vi "AuthenticationTest.vi"(8 "error in (no error)":errorcluster) -> (0 "error out":errorcluster, 3 "Match?":bool)   [LabVIEW 2016, in "User Interface.lvlib"]
uses:
  User Interface.lvlib
  Authentication State.ctl
  Database/Database.lvlib
  Database/Class/DB/Credential.ctl
  Action log.ctl
panel:
  out "Time 2":string="Authentication"
  out "Msg Out":string
  in  "Password":string
  in  "Username":string(combo)
  in  "User Level":string(combo)
  in  "Cancel":bool
  in  "Delete":bool
  in  "Add":bool
  in  "Edit":bool
  in  "Authentication Tab":enum32{"User", "Edit User"}(tab)
  in  "User Name":string(combo)
  in  "Password":string
  in  "Log":bool
  out "Time":string="Sat  8/3/2019  8:10:44 PM"
  in  "Update":bool
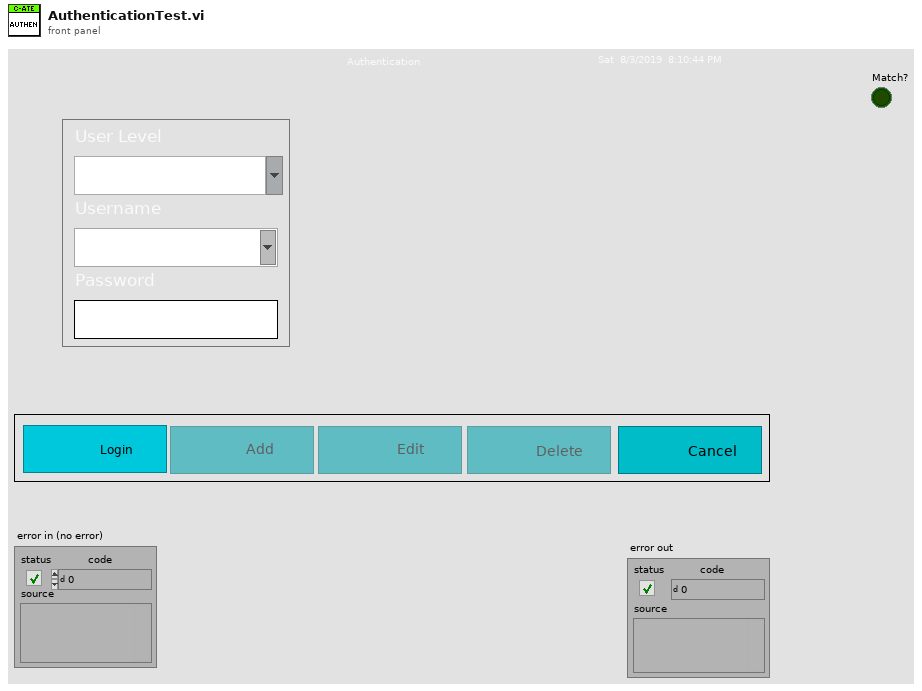
[diagram p1: front panel]
types:
  T1 = typedef "User Interface.lvlib/Authentication State.ctl" = enum16{"Initialize", "Main", "Add User", "Delete User", "Close"}
  T2 = typedef "User Interface.lvlib/Action log.ctl" = enum16{"Init", "Read", "Write", "Close"}
  T3 = typedef "Database.lvlib/Credential.ctl" = cluster{"User Level":string, "User Name":string, "Password":string}
  T4 = enum8{"Enabled", "Disabled", "Disabled and Grayed Out"}
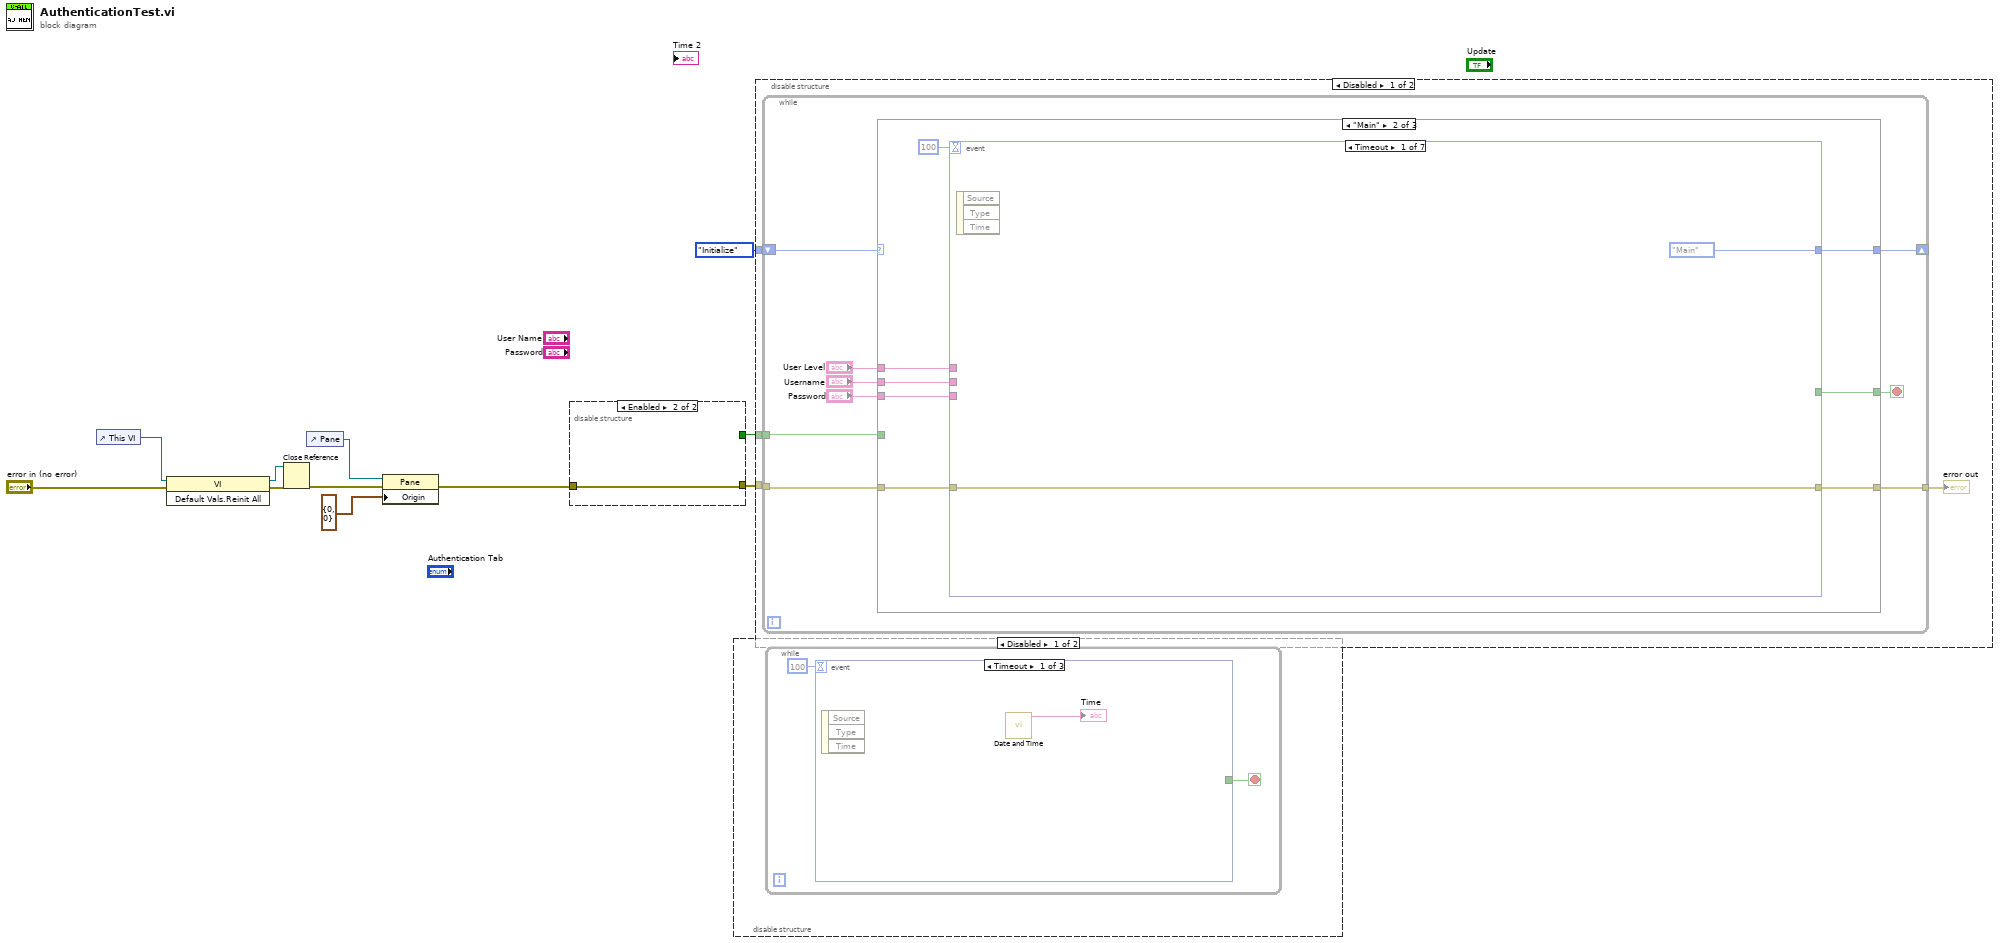
[diagram p0: block diagram]
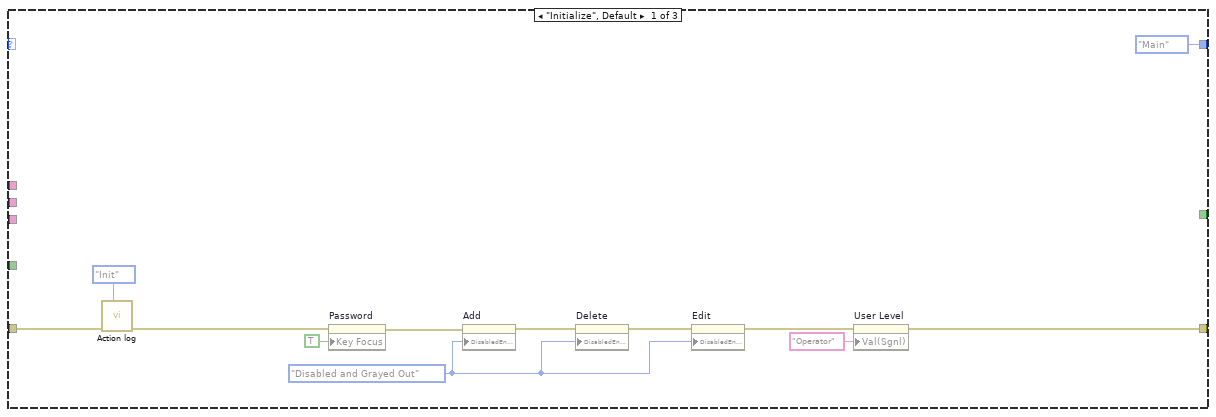
[diagram p2: hidden frame]
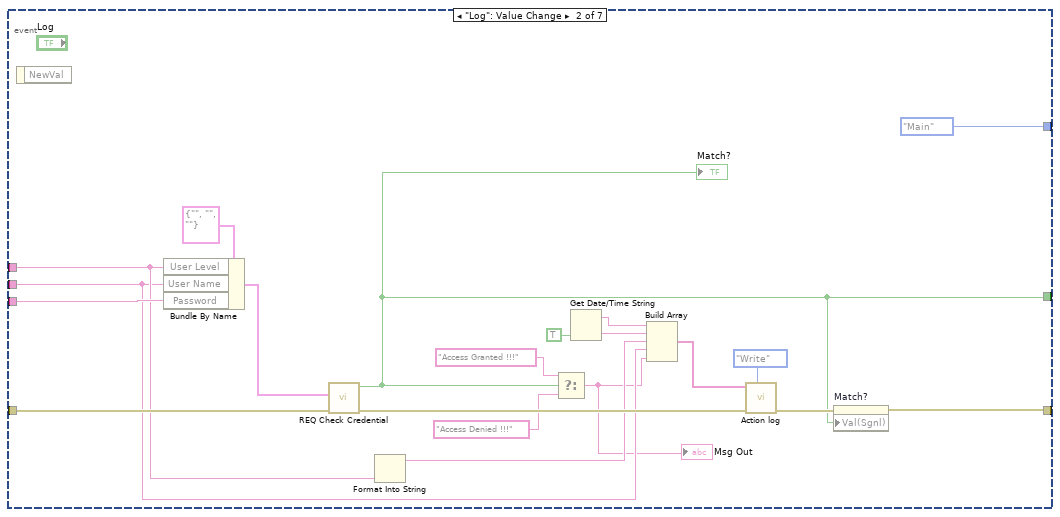
[diagram p3: hidden frame]
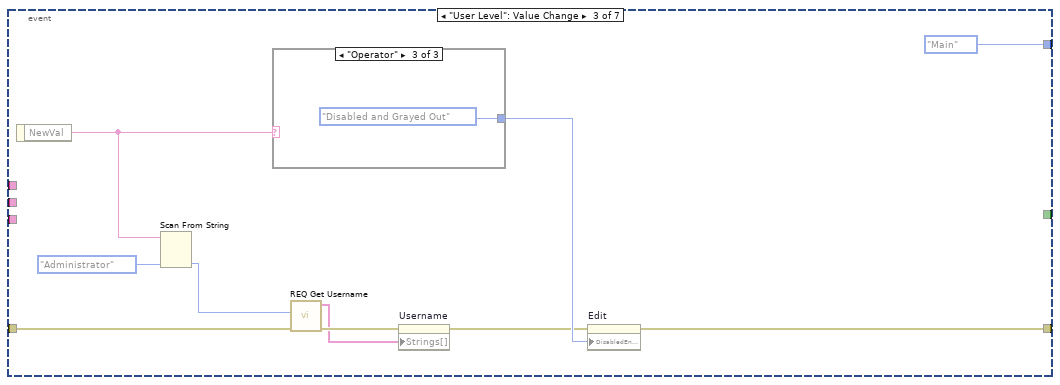
[diagram p4: hidden frame]
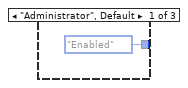
[diagram p5: hidden frame]
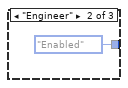
[diagram p6: hidden frame]
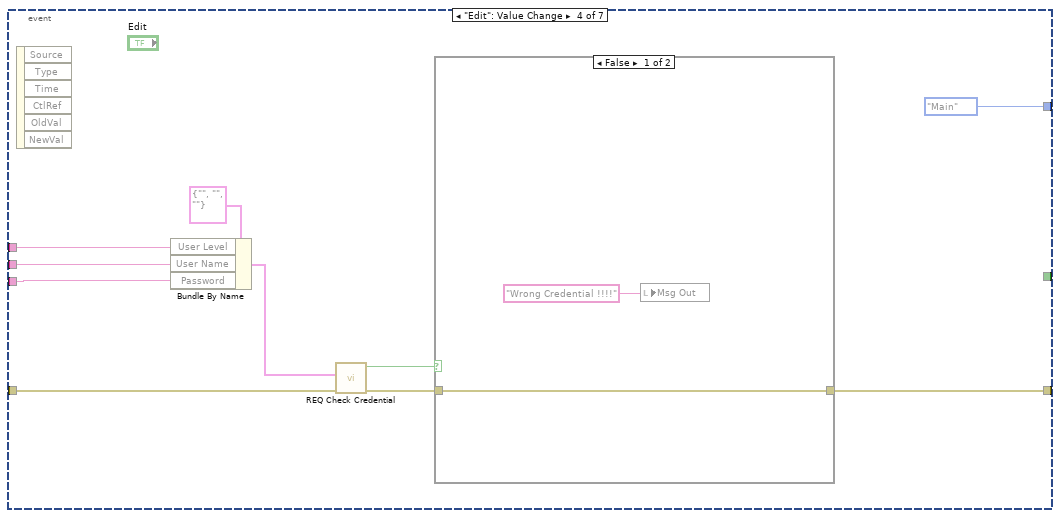
[diagram p7: hidden frame]
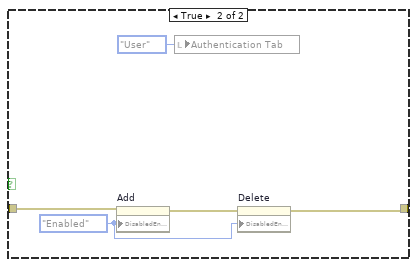
[diagram p8: hidden frame]
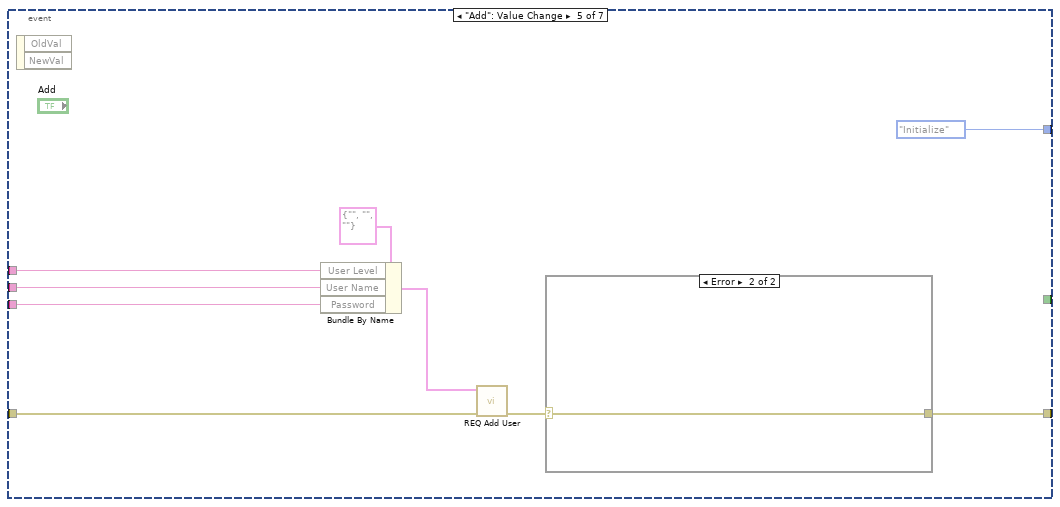
[diagram p9: hidden frame]
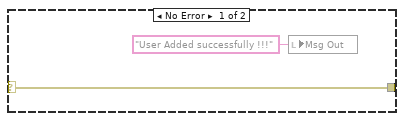
[diagram p10: hidden frame]
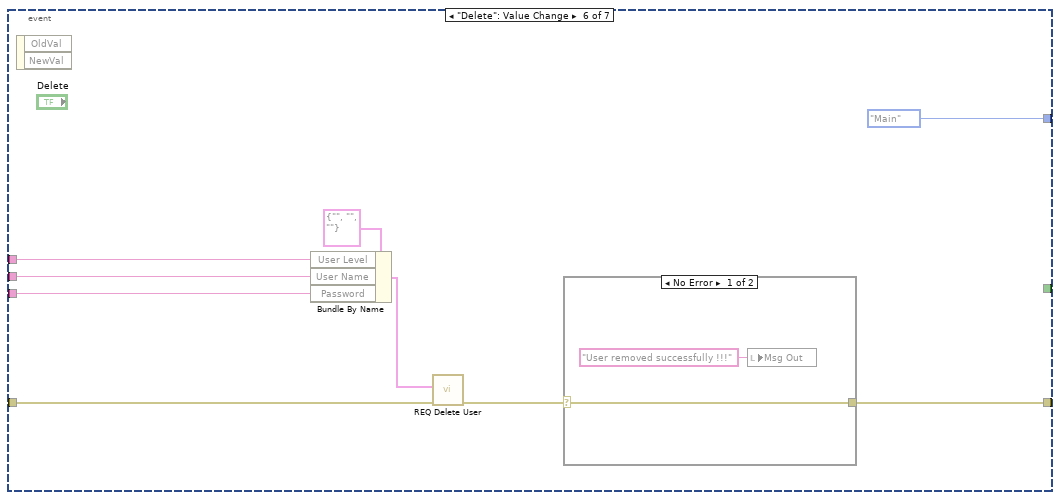
[diagram p11: hidden frame]
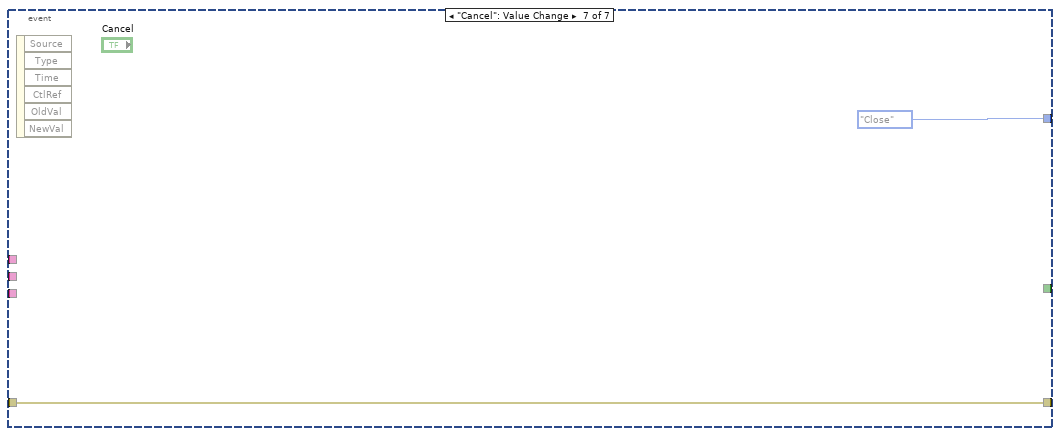
[diagram p13: hidden frame]
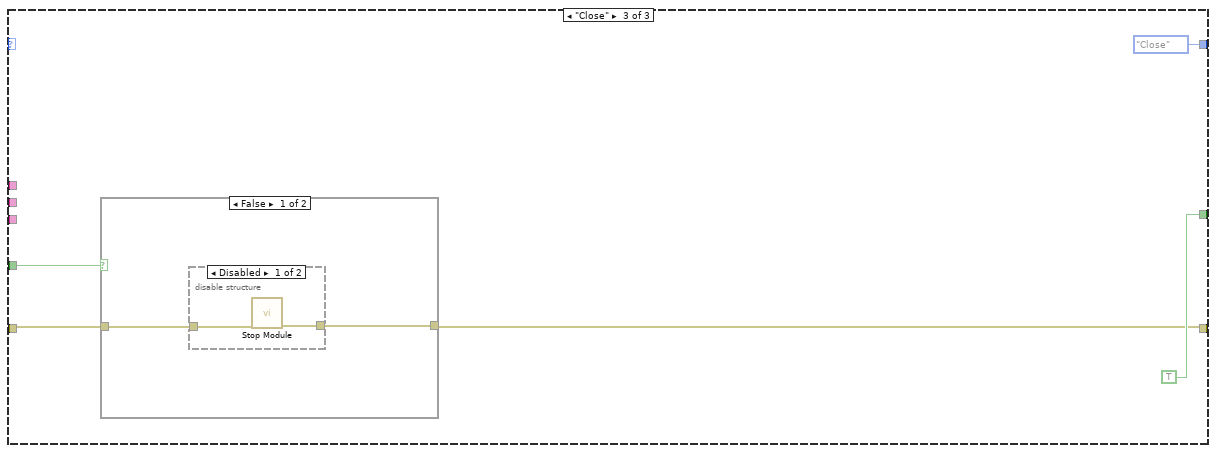
[diagram p14: hidden frame]
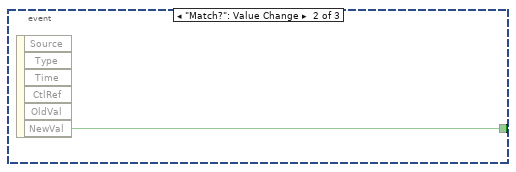
[diagram p18: hidden frame]
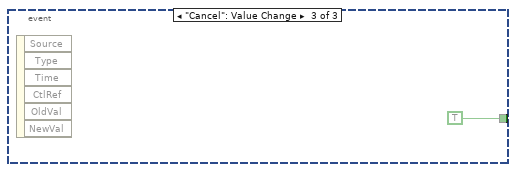
[diagram p19: hidden frame]
diagram:
  n1 = control-ref of="This VI"() -> (w10:refnum<vi>)
  n2 = invoke class="VI" method="Default Vals.Reinit All"(reference=w10, error in="error in (no error)") -> (reference out=w8:refnum<vi>, error out=w9:errorcluster)  [unwired: 1 in, 1 out]
  n3 = Close Reference(reference=w8, error in (no error)=w9) -> (error out=w7:errorcluster)
  n4 = control-ref of="Pane"() -> (w4:refnum<vi>)
  n5 = property class="Pane"(reference=w4, error in=w7, "Origin"=cluster{"Horizontal":i16, "Verticle":i16} {"Horizontal"=0, "Verticle"=0} ("Origin (0,0)")) -> (error out=w3:errorcluster)  [unwired: 1 out]
  n6 = disable-structure shown="Enabled" {
    disable-tunnel: w3 -> [w14 w17]
    disable-tunnel: [w13 w17] -> w2
    disable-tunnel: [w12 _] -> w1
    frame Disabled {
      n7 = call "Start Module.vi"("error in"=w14) -> ("error out"=w15:errorcluster, "Wait for Event Sync?"=w16:bool, "Module Was Already Running?"=w12:bool)  [unwired: 7 in, 1 out]
      n8 = call "Synchronize Module Events.vi"("error in"=w15, "Wait for Event Sync?"=w16) -> ("error out"=w13:errorcluster)  [unwired: 9 in]
    }
    frame Enabled {
    }
  }
  n9 = disable-structure shown="Disabled" {
    frame Disabled {
      n10 = while {
        stop <- w18 stop-if-true
        n11 = event shown="[0] Timeout" {
          selector: _ -> [_ _ _]
          dyn-events: _ -> [_ _ _]
          timeout: 100 -> [_ _ _]
          tunnel: [_ w21 TRUE] -> w18
          event Timeout {
            n12 = event-data() -> ()  [unwired: 1 in, 3 out]
            n13 = call "Date and Time.vi"() -> ("Current Time"=→"Time":string)  [unwired: 11 in]
          }
          event "Match?": Value Change {
            n14 = event-data() -> ("NewVal"=w21:bool)  [unwired: 1 in, 5 out]
          }
          event "Cancel": Value Change {
            n15 = event-data() -> ()  [unwired: 1 in, 6 out]
          }
        }
      }
    }
    frame Enabled {
    }
  }
  n16 = disable-structure shown="Disabled" {
    disable-tunnel: Authentication_State."Initialize" -> [w26 _]
    disable-tunnel: w2 -> [w24 _]
    disable-tunnel: w1 -> [w23 _]
    frame Disabled {
      n17 = while {
        shift-right: [w32] -> _
        shift-left: w26 -> [w35]
        tunnel: w24 -> [w34]
        tunnel: [w33] -> w25
        tunnel: w23 -> [w30]
        stop <- w31 stop-if-true
        n18 = case shown="\"Main\"" w35 {
          tunnel: w34 -> [w41 w55 w135]
          tunnel: [w37 w53 w134] -> w33
          tunnel: [Authentication_State."Main" w54 Authentication_State."Close"] -> w32
          tunnel: [_ w48 TRUE] -> w31
          tunnel: "User Level" -> [_ w51 _]
          tunnel: "Username" -> [_ w50 _]
          tunnel: "Password" -> [_ w49 _]
          tunnel: w30 -> [_ _ w136]
          frame "Initialize", Default {
            w44 = T4."Disabled and Grayed Out" ("Disabled")
            n19 = call "Action log.vi"("Command"=Action_log."Init", "error in (no error)"=w41) -> ("error out"=w39:errorcluster)  [unwired: 9 in]
            n20 = property on="Password" class="Str"(error in=w39, "Key Focus"=TRUE) -> (error out=w42:errorcluster)  [unwired: 1 in, 1 out]
            n21 = property on="Add" class="Bool"(error in=w42, "DisabledEnum"=w44) -> (error out=w46:errorcluster)  [unwired: 1 in, 1 out]
            n22 = property on="Delete" class="Bool"(error in=w46, "DisabledEnum"=w44) -> (error out=w45:errorcluster)  [unwired: 1 in, 1 out]
            n23 = property on="Edit" class="Bool"(error in=w45, "DisabledEnum"=w44) -> (error out=w38:errorcluster)  [unwired: 1 in, 1 out]
            n24 = property on="User Level" class="CmbBox"(error in=w38, "Val(Sgnl)"="Operator" ("Value (Signaling)")) -> (error out=w37:errorcluster)  [unwired: 1 in, 1 out]
          }
          frame "Main" {
            n25 = event shown="[0] Timeout" {
              selector: _ -> [_ _ _ _ _ _ _]
              dyn-events: _ -> [_ _ _ _ _ _ _]
              timeout: 100 -> [_ _ _ _ _ _ _]
              tunnel: w55 -> [w56 w77 w85 w97 w115 w125 w132]
              tunnel: [Authentication_State."Main" Authentication_State."Main" Authentication_State."Main" Authentication_State."Main" Authentication_State."Initialize" Authentication_State."Main" Authentication_State."Close"] -> w54
              tunnel: [w56 w59 w84 w91 w108 w120 w132] -> w53
              tunnel: w51 -> [_ w67 _ w96 w112 w124 _]
              tunnel: w50 -> [_ w62 _ w95 w111 w123 _]
              tunnel: w49 -> [_ w75 _ w94 w110 w122 _]
              tunnel: [_ w58 _ _ _ _ _] -> w48
              event Timeout {
                n26 = event-data() -> ()  [unwired: 1 in, 3 out]
              }
              event "Log": Value Change {
                n27 = event-data() -> ()  [unwired: 1 in, 1 out]
                n28 = Bundle By Name(cluster=T3 {"User Level"="", "User Name"="", "Password"=""} ("Credential"), "User Level"=w67, "User Name"=w62, "Password"=w75) -> (w73:T3)
                n29 = call "REQ Check Credential.vi"("error in"=w77, "Credential"=w73) -> ("error out"=w71:errorcluster, "Match?"=w58:bool)  [unwired: 7 in, 1 out]
                "Match?" <- w58
                n30 = Format Into String(w67) -> (resulting string=w63:string)  [unwired: 3 in, 1 out]
                n31 = Select(t="Access Granted !!!", s=w58, f="Access Denied !!!") -> (s? t:f=w61:string)
                "Msg Out" <- w61
                n32 = Get Date/Time String(want seconds? (F)=TRUE) -> (date string=w69:string, time string=w68:string)  [unwired: 2 in]
                n33 = Build Array(w69, w68, w63, w62, w61) -> (w64:string[])
                n34 = call "Action log.vi"("Command"=Action_log."Write", "error in (no error)"=w71, "Data"=w64) -> ("error out"=w60:errorcluster)  [unwired: 8 in]
                n35 = property on="Match?" class="Bool (strict)"(error in=w60, "Val(Sgnl)"=w58) -> (error out=w59:errorcluster)  [unwired: 1 in, 1 out]
              }
              event "User Level": Value Change {
                n36 = event-data() -> ("NewVal"=w82:string)  [unwired: 1 in]
                n37 = Scan From String(input string=w82, default 1=enum16{"Administrator", "Engineer", "Operator"}."Administrator" ("User Level")) -> (output 1=w81:enum16{"Administrator", "Engineer", "Operator"})  [unwired: 3 in, 3 out]
                n38 = case shown="\"Operator\"" w82 {
                  tunnel: [T4."Enabled" ("Disabled") T4."Enabled" ("Disabled") T4."Disabled and Grayed Out" ("Disabled")] -> w86
                  frame "Administrator", Default {
                  }
                  frame "Engineer" {
                  }
                  frame "Operator" {
                  }
                }
                n39 = call "REQ Get Username.vi"("error in"=w85, "User Level"=w81) -> ("error out"=w80:errorcluster, "Username"=w78:string[])  [unwired: 7 in, 1 out]
                n40 = property on="Username" class="CmbBox"(error in=w80, "Strings[]"=w78) -> (error out=w79:errorcluster)  [unwired: 1 in, 1 out]
                n41 = property on="Edit" class="Bool"(error in=w79, "DisabledEnum"=w86) -> (error out=w84:errorcluster)  [unwired: 1 in, 1 out]
              }
              event "Edit": Value Change {
                n42 = event-data() -> ()  [unwired: 1 in, 6 out]
                n43 = Bundle By Name(cluster=T3 {"User Level"="", "User Name"="", "Password"=""} ("Credential"), "User Level"=w96, "User Name"=w95, "Password"=w94) -> (w98:T3)
                n44 = call "REQ Check Credential.vi"("error in"=w97, "Credential"=w98) -> ("error out"=w92:errorcluster, "Match?"=w93:bool)  [unwired: 7 in, 1 out]
                n45 = case shown="False" w93 {
                  tunnel: w92 -> [w102 w104]
                  tunnel: [w102 w103] -> w91
                  frame False {
                    n46 = local write "Msg Out"("Wrong Credential !!!!" ("message")) -> ()
                  }
                  frame True {
                    w105 = T4."Enabled" ("Disabled")
                    n47 = property on="Add" class="Bool"(error in=w104, "DisabledEnum"=w105) -> (error out=w106:errorcluster)  [unwired: 1 in, 1 out]
                    n48 = local write "Authentication Tab"(enum32{"User", "Edit User"}."User" ("Authentication Tab")) -> ()
                    n49 = property on="Delete" class="Bool"(error in=w106, "DisabledEnum"=w105) -> (error out=w103:errorcluster)  [unwired: 1 in, 1 out]
                  }
                }
              }
              event "Add": Value Change {
                n50 = event-data() -> ()  [unwired: 1 in, 2 out]
                n51 = Bundle By Name(cluster=T3 {"User Level"="", "User Name"="", "Password"=""} ("Credential"), "User Level"=w112, "User Name"=w111, "Password"=w110) -> (w113:T3)
                n52 = call "REQ Add User.vi"("error in"=w115, "Credential"=w113) -> ("error out"=w109:errorcluster)  [unwired: 9 in]
                n53 = case shown="Error" w109 {
                  selector: w109 -> [w117 w119]
                  tunnel: [w117 w119] -> w108
                  frame No Error {
                    n54 = local write "Msg Out"("User Added successfully !!!" ("Msg Out")) -> ()
                  }
                  frame Error {
                  }
                }
              }
              event "Delete": Value Change {
                n55 = event-data() -> ()  [unwired: 1 in, 2 out]
                n56 = Bundle By Name(cluster=T3 {"User Level"="", "User Name"="", "Password"=""} ("Credential"), "User Level"=w124, "User Name"=w123, "Password"=w122) -> (w126:T3)
                n57 = call "REQ Delete User.vi"("error in"=w125, "Credential"=w126) -> ("error out"=w121:errorcluster)  [unwired: 9 in]
                n58 = case shown="No Error" w121 {
                  selector: w121 -> [w129 w131]
                  tunnel: [w129 w131] -> w120
                  frame No Error {
                    n59 = local write "Msg Out"("User removed successfully !!!" ("Msg Out")) -> ()
                  }
                  frame Error {
                  }
                }
              }
              event "Cancel": Value Change {
                n60 = event-data() -> ()  [unwired: 1 in, 6 out]
              }
            }
          }
          frame "Close" {
            n61 = case shown="False" w136 {
              tunnel: w135 -> [w140 w143]
              tunnel: [w139 w143] -> w134
              frame False {
                n62 = disable-structure shown="Disabled" {
                  disable-tunnel: w140 -> [w142 _]
                  disable-tunnel: [w141 _] -> w139
                  frame Disabled {
                    n63 = call "Stop Module.vi"("error in"=w142) -> ("error out"=w141:errorcluster)  [unwired: 10 in]
                  }
                  frame Enabled {
                  }
                }
              }
              frame True {
              }
            }
          }
        }
      }
      "error out" <- w25
    }
    frame Enabled {
    }
  }
